vi "WSVCAP SHL Host LL Set Write Data Parameter.vi"(0 "Write Byte In":u64, 11 "error in (no error)":errorcluster) -> (15 "error out":errorcluster)   [LabVIEW 2012]
uses:
  Type Defs/WSVCAP SHL Top Level Control Operation Enum.ctl
  Type Defs/WSVCAP SHL Top Level Control Enum.ctl
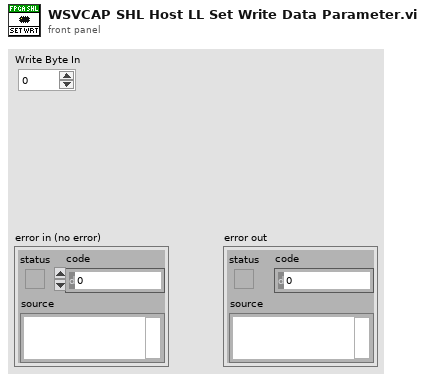
[diagram p1: front panel]
types:
  T1 = typedef "WSVCAP SHL Top Level Control Enum.ctl" = enum16{"Start", "Cmd", "Transaction", "Wait Ticks", "Socket Mask", "UUT Set", "Slave Address", "Sub Address", "Bytes to Write", "Bytes to Read", "Write Data", "Write Flag", "Read Data", "Read Flag", "Ack Read", "Read Status Flag", "Ack Read Status", "Status", "Cycle Count", "Stop Cycle", "Exit"}
  T2 = typedef "WSVCAP SHL Top Level Control Operation Enum.ctl" = enum16{"Initialize", "Set Control", "Read Control", "Close"}
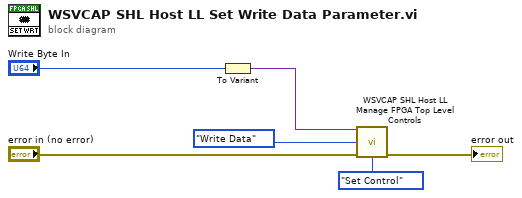
[diagram p0: block diagram]
diagram:
  n1 = To Variant(anything="Write Byte In") -> (Variant=w2:variant)
  n2 = call "WSVCAP SHL Host LL Manage FPGA Top Level Controls.vi"("Value In"=w2, "FPGA Top Level Control"=WSVCAP_SHL_Top_Level_Control_Enum."Write Data", "error in (no error)"="error in (no error)", "Operation"=WSVCAP_SHL_Top_Level_Control_Operation_Enum."Set Control") -> ("error out"=→"error out":errorcluster)  [unwired: 10 in, 1 out]
